vi "Read ADS1015 ADC Driver.vi"(8 "error in (no error)":errorcluster, 11 "LINX-AutomationHat in":refnum<class "LINX-AutomationHat.lvclass">) -> (0 "error out":errorcluster, 2 "LINX-ADS1X15":refnum<class "LINX-ADS1X15.lvclass">, 3 "LINX-AutomationHat out":refnum<class "LINX-AutomationHat.lvclass">)   [LabVIEW 2020, in "LINX-AutomationHat.lvclass"]
uses:
  LINX-AutomationHat.lvclass
  LINX-ADS1015/LINX-ADS1X15.lvclass
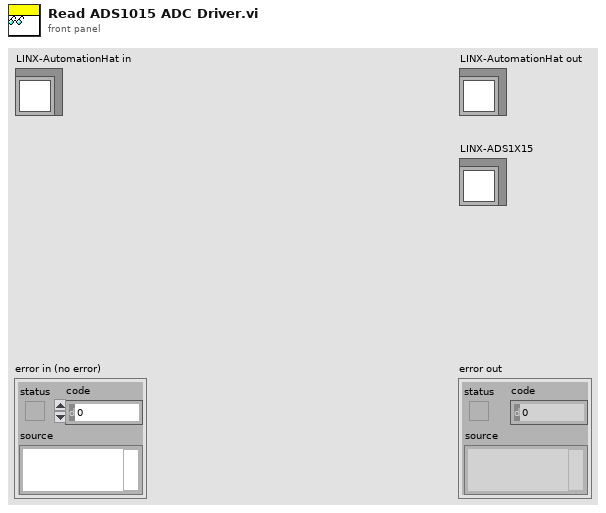
[diagram p1: front panel]
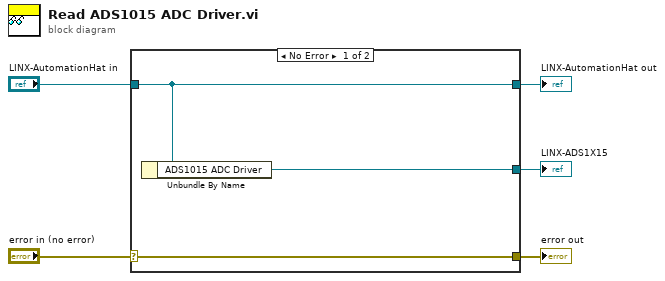
[diagram p0: block diagram]
diagram:
  n1 = case shown="No Error" "error in (no error)" {
    selector: "error in (no error)" -> [w8 w9]
    tunnel: [w8 w9] -> w4
    tunnel: [w7 w10] -> w2
    tunnel: "LINX-AutomationHat in" -> [w7 w10]
    tunnel: [w6 _] -> w1
    frame No Error {
      n2 = Unbundle By Name(w7) -> ("ADS1015 ADC Driver"=w6:refnum<class "LINX-ADS1X15.lvclass">)
    }
    frame Error {
    }
  }
  "error out" <- w4
  "LINX-AutomationHat out" <- w2
  "LINX-ADS1X15" <- w1
